vi "Add Permission.vi"(8 "error in (no error)":errorcluster, 9 "Permissions":T1[](array[typedef]), 10 "Label":string, 11 "Topic":refnum<class "Topic.lvclass">) -> (0 "error out":errorcluster, 3 "Topic out":refnum<class "Topic.lvclass">)   [LabVIEW 2015, in "NI_AWS_SNS.lvlib" / "Topic.lvclass"]
doc: "Adds a statement to a topic's access control policy, granting access for the specified AWS accounts to the specified actions."
uses:
  Topic.lvclass
  Permission.ctl
  Action Name.ctl
  Core/HTTP Request/Request Options.ctl
  Core/HTTP Request/Name Value Pair.ctl
  Core/HTTP Request/Region handling.ctl
  Core/HTTP Request/URL formatting.ctl
  Core/ARN/ARN.lvclass/ARN.ctl
  Core/ARN/Read ARN.vi
  Core/HTTP Request/HTTP Request.lvclass
  NI_AWS_SNS.lvlib
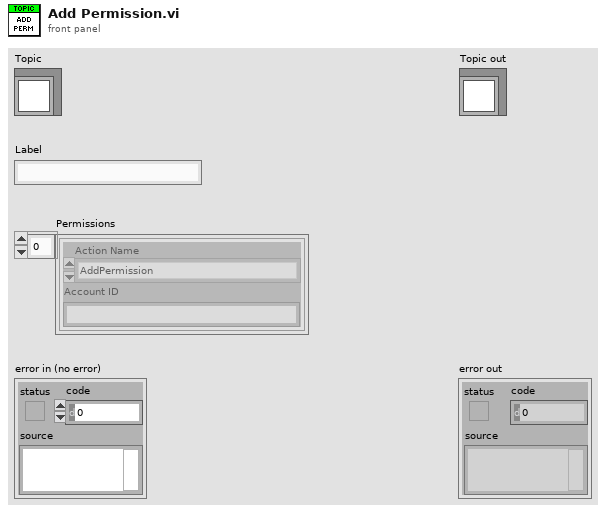
[diagram p1: front panel]
types:
  T1 = typedef "NI_AWS_SNS.lvlib/Topic.lvclass/Permission.ctl" = cluster{"Action Name":T2, "Account ID":string}
  T2 = typedef "NI_AWS_SNS.lvlib/Action Name.ctl" = enum16{"AddPermission", "CheckIfPhoneNumberIsOptedOut", "ConfirmSubscription", "CreatePlatformApplication", "CreatePlatformEndpoint", "CreateTopic", "DeleteEndpoint", "DeletePlatformApplication", "DeleteTopic", "GetEndpointAttributes", "GetPlatformApplicationAttributes", "GetSMSAttributes", "GetSubscriptionAttributes", "GetTopicAttributes", "ListEndpointsByPlatformApplication", "ListPhoneNumbersOptedOut", "ListPlatformApplications", "ListSubscriptions", "ListSubscriptionsByTopic", "ListTopics", "OptInPhoneNumber", "Publish", "RemovePermission", "SetEndpointAttributes", "SetPlatformApplicationAttributes", "SetSMSAttributes", "SetSubscriptionAttributes", "SetTopicAttributes", "Subscribe", "Unsubscribe"}
  T3 = typedef "NI_AWS_Core.lvlib/HTTP Request.lvclass/Name Value Pair.ctl" = cluster{"name":string, "value":string}
  T4 = typedef "NI_AWS_Core.lvlib/HTTP Request.lvclass/Request Options.ctl" = cluster{"request headers":T3[], "request parameters":T3[], "request body":string, "region handling":T5, "URL formatting":T6}
  T5 = typedef "NI_AWS_Core.lvlib/HTTP Request.lvclass/Region handling.ctl" = enum16{"use region everywhere", "use region (authentication only)", "use region (URL only)", "ignore region everwhere"}
  T6 = typedef "NI_AWS_Core.lvlib/HTTP Request.lvclass/URL formatting.ctl" = enum16{"region-", "region."}
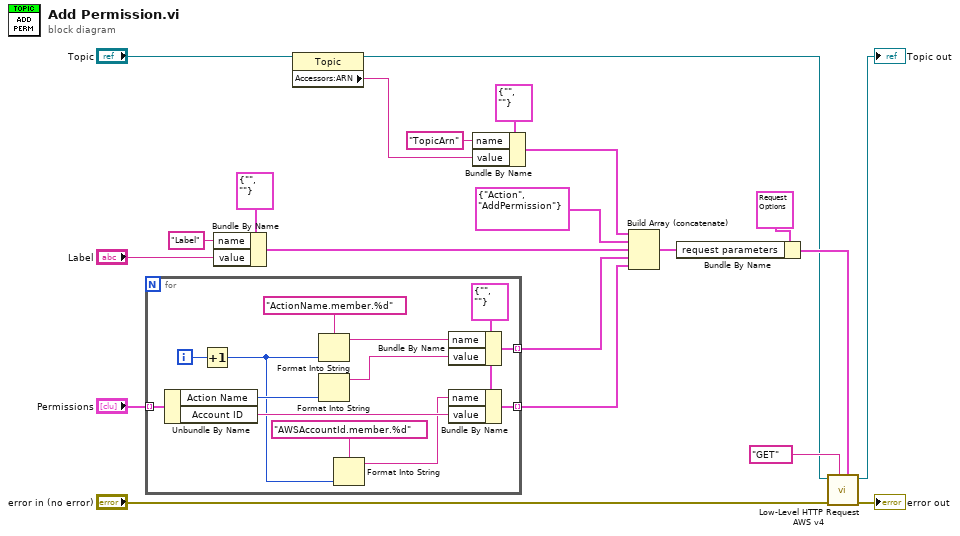
[diagram p0: block diagram]
diagram:
  n1 = for {
    tunnel: "Permissions" -> [w34] mode=indexing
    tunnel: [w32] -> w6 mode=indexing
    tunnel: [w31] -> w5 mode=indexing
    i -> [w30]
    w33 = T3 {"name"="", "value"=""} ("element")
    n2 = Unbundle By Name(w34) -> ("Action Name"=w27:T2, "Account ID"=w25:string)
    n3 = Increment(x=w30) -> (x+1=w23:i32)
    n4 = Format Into String(format string="ActionName.member.%d", w23) -> (resulting string=w28:string)  [unwired: 2 in, 1 out]
    n5 = Format Into String(w27) -> (resulting string=w26:string)  [unwired: 3 in, 1 out]
    n6 = Format Into String(format string="AWSAccountId.member.%d", w23) -> (resulting string=w22:string)  [unwired: 2 in, 1 out]
    n7 = Bundle By Name(cluster=w33, "name"=w28, "value"=w26) -> (w32:T3)
    n8 = Bundle By Name(cluster=w33, "name"=w22, "value"=w25) -> (w31:T3)
  }
  n9 = Bundle By Name(cluster=T3 {"name"="", "value"=""} ("element"), "name"="Label", "value"="Label") -> (w8:T3)
  n10 = property class="Topic"(reference="Topic") -> (reference out=w1:refnum<class "Topic.lvclass">, "Accessors:ARN"=w13:string)  [unwired: 1 in, 1 out]
  n11 = Bundle By Name(cluster=T3 {"name"="", "value"=""} ("element"), "name"="TopicArn", "value"=w13) -> (w12:T3)
  n12 = Build Array (concatenate)(w12, T3 {"name"="Action", "value"="AddPermission"} ("Cluster"), w8, w6, w5) -> (w16:T3[])
  n13 = Bundle By Name(cluster=T4 {"request headers"=[], "request parameters"=[{"name"="Action", "value"="ListQueues"}], "request body"="", "region handling"=enum."use region everywhere", "URL formatting"=enum."region."} ("Request Options"), "request parameters"=w16) -> (w3:T4)
  n14 = call "Low-Level HTTP Request AWS v4.vi"("Request Options"=w3, "HTTP-Verb"="GET", "error in (no error)"="error in (no error)", "AWS Core in"=w1) -> ("error out"=→"error out":errorcluster, "AWS Core out"=→"Topic out":refnum<class "Topic.lvclass">)  [unwired: 4 in, 2 out]
